vi "IC_Clear.vi"(1 "ICImagingControl 2":refnum<k7>) -> (0 "ICImagingControl":refnum<k7>)   [LabVIEW 2020]
doc: "This VI stops a may be runnig live video stream. It removes frame filters from the devices path and closes the current video capture device.\nIt should be inserted at the beginning of a VI and when it ends to keep IC Imaging Control clean."
uses:
  <vilib>/Utility/error.llb/DialogType.ctl
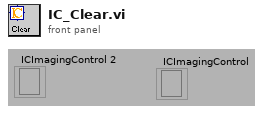
[diagram p1: front panel]
types:
  T1 = typedef "DialogType.ctl" = u16
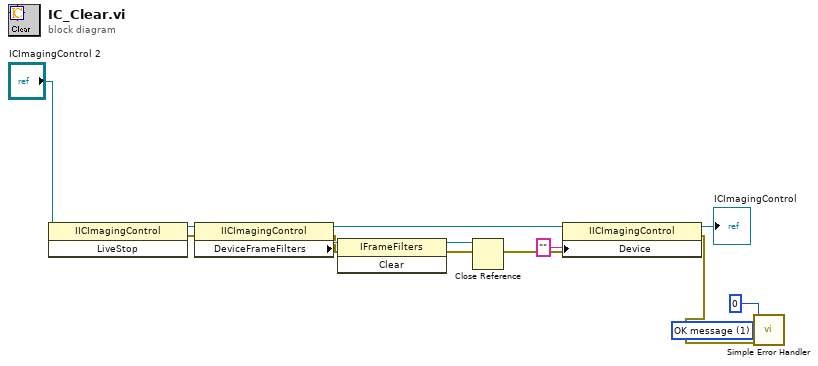
[diagram p0: block diagram]
diagram:
  w2 = T1 1 items=["no dialog", "OK message", "continue or stop message", "OK message + warnings", "continue/stop + warnings"] ("type of dialog (OK msg:1)")
  n1 = invoke class="IICImagingControl" method="LiveStop"(reference="ICImagingControl 2") -> (reference out=w8:refnum<k7>, error out=w6:errorcluster)  [unwired: 2 in, 1 out]
  n2 = property class="IICImagingControl"(reference=w8, error in=w6) -> (reference out=w11:refnum<k7>, error out=w5:errorcluster, "DeviceFrameFilters"=w9:refnum<k7>)
  n3 = invoke class="IFrameFilters" method="Clear"(reference=w9, error in=w5) -> (reference out=w10:refnum<k7>, error out=w4:errorcluster)  [unwired: 1 in, 1 out]
  n4 = Close Reference(reference=w10) -> ()  [unwired: 1 in, 1 out]
  n5 = property class="IICImagingControl"(reference=w11, error in=w4, "Device"="") -> (reference out=→"ICImagingControl":refnum<k7>, error out=w1:errorcluster)
  n6 = call <vilib>:"Simple Error Handler.vi"("error code (no error:0)"=0, "type of dialog (OK msg:1)"=w2, "error in (no error)"=w1) -> ()  [unwired: 2 in, 5 out]
